vi "Pockels Cal_Eliminate empty objectives.vi"(11 "New cal section":string[][](array[string])) -> (3 "New cal section":string[][](array[string]))   [LabVIEW 2013]
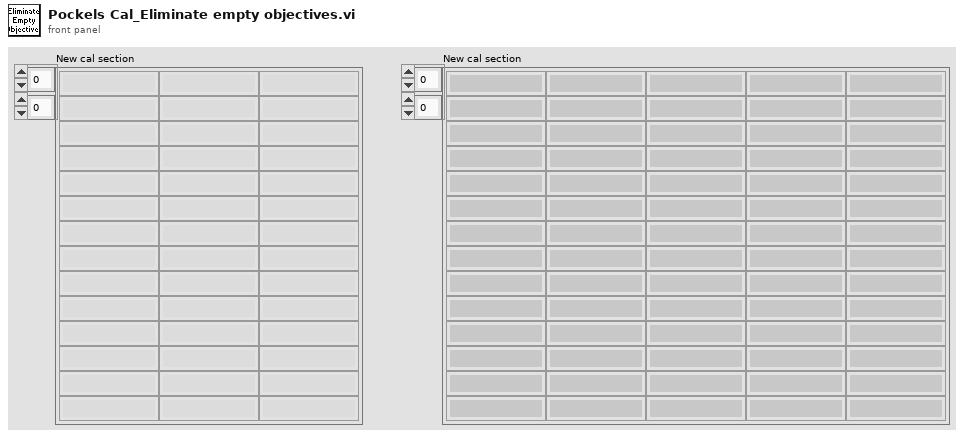
[diagram p1: front panel]
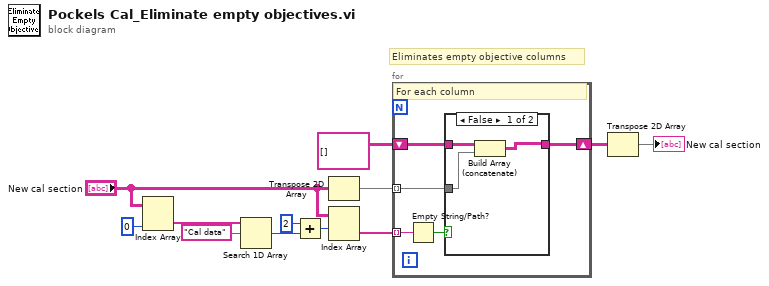
[diagram p0: block diagram]
diagram:
  # "Eliminates empty objective columns"
  n1 = Index Array(array="New cal section", index (col)=0 ("disabled index (col)")) -> (element=w1:string[])  [unwired: 1 in]
  n2 = Search 1D Array(1D array=w1, element="Cal data") -> (index of element=w3:i32)  [unwired: 1 in]
  n3 = Add(x=2, y=w3) -> (x+y=w5:i32)
  n4 = Transpose 2D Array(2D array="New cal section") -> (transposed array=w9:string[][])
  n5 = Index Array(array="New cal section", index (row)=w5) -> (element=w8:string[])  [unwired: 1 in]
  n6 = for {
    tunnel: w9 -> [w13] mode=indexing
    tunnel: w8 -> [w17] mode=indexing
    shift-right: [w14] -> w11
    shift-left: string[][] [] ("New cal section") -> [w15]
    # "For each column"
    n7 = Empty String/Path?(string/path=w17) -> (empty?=w16:bool)
    n8 = case shown="False" w16 {
      tunnel: [w19 w21] -> w14
      tunnel: w15 -> [w20 w21]
      tunnel: w13 -> [w18 _]
      frame False {
        n9 = Build Array (concatenate)(w20, w18) -> (w19:string[][])
      }
      frame True {
      }
    }
  }
  n10 = Transpose 2D Array(2D array=w11) -> (transposed array=→"New cal section":string[][])
